vi "New.vi"(4 "Plugin":refnum<class "Plugin.lvclass">, 5 "thread base name":string="untitled", 6 "Logging Interface":refnum<class "Logging Interface.lvclass">, 7 "Plugin Interfaces Pool":refnum<class "Plugin Interface Pool.lvclass">, 8 "error in (no error)":errorcluster, 9 "Transfer Groups":refnum<class "Transfer Group.lvclass">[](array[class]), 10 "thread configuration":T1={"buffer converter settings"=[], "transceiver settings"=[], "custom settings"=[], "processor"=-2, "priority offset"=0}, 11 "Plugin Thread type":refnum<class "Plugin Thread.lvclass">) -> (0 "error out":errorcluster, 2 "Plugin Thread Interface":refnum<class "Plugin Interface.lvclass">, 3 "Plugin Thread out":refnum<class "Plugin Thread.lvclass">)   [LabVIEW 2017, in "DSF Core.lvlib" / "Plugin Thread.lvclass"]
uses:
  Thread/Plugin/Plugin Thread.lvclass
  C:/Git/DSF/Core/Classes/Thread/Thread.lvclass
  Transfer Group/Transfer Group.lvclass
  Pool/Plugin Interface/Plugin Interface Pool.lvclass
  Interface/Plugin/Plugin Interface.lvclass
  C:/Git/DSF/Core/Classes/Interface/Interface.lvclass
  Typedefs/DSF Engine Plugin Thread Configuration.ctl
  Typedefs/DSF Settings Info.ctl
  Interface/Logging/Logging Interface.lvclass
  Plugin/Plugin.lvclass
  Thread/Thread Settings.ctl
  Thread/Plugin/Plugin Thread.lvclass/Plugin Thread.ctl
  Thread/Thread.lvclass
  Interface/Interface.lvclass
  Timing/Timing.lvclass
  DSF Core.lvlib
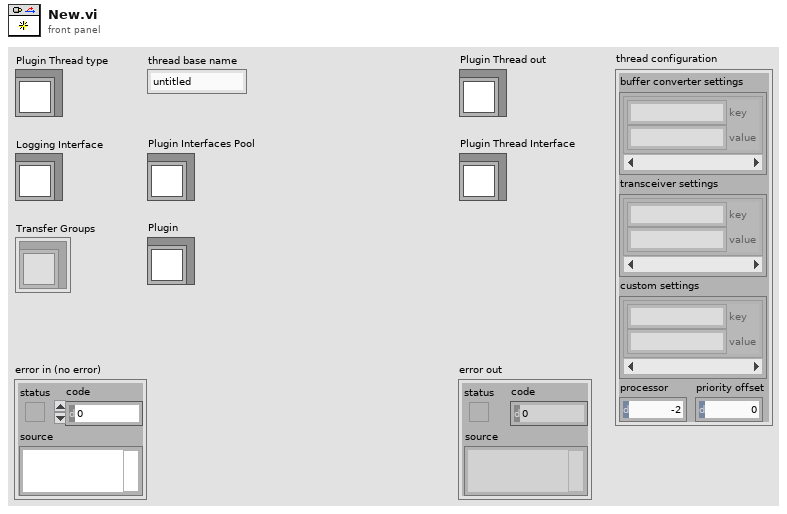
[diagram p1: front panel]
types:
  T1 = typedef "DSF Core.lvlib/DSF Engine Plugin Thread Configuration.ctl" = cluster{"buffer converter settings":T2, "transceiver settings":T2, "custom settings":T2, "processor":i32, "priority offset":i16}
  T2 = typedef "DSF Core.lvlib/DSF Settings Info.ctl" = cluster{"key":string, "value":string}[]
  T3 = typedef "DSF Core.lvlib/Thread.lvclass/Thread Settings.ctl" = cluster{"Priority":u16, "Processor":i32, "ID":i32}
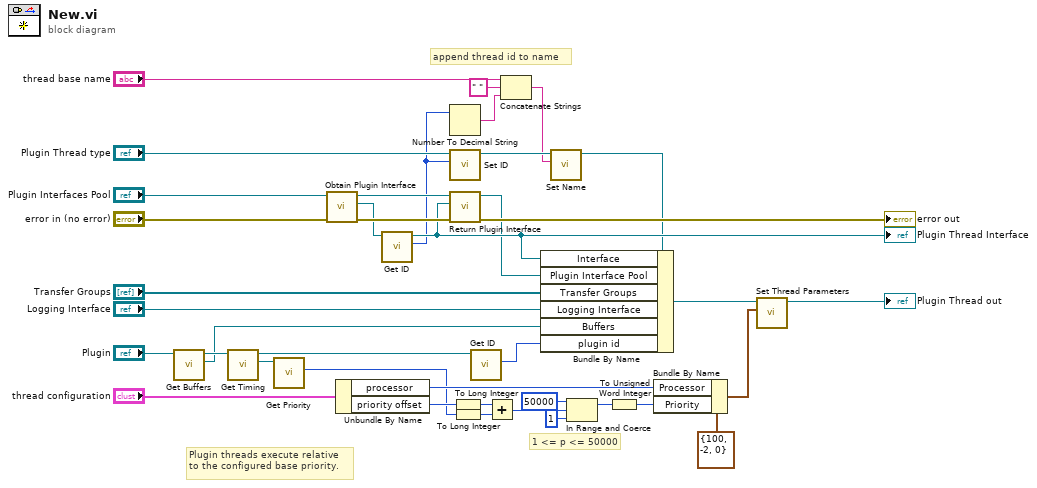
[diagram p0: block diagram]
diagram:
  # "1 <= p <= 50000"
  # "append thread id to name"
  # "Plugin threads execute relative to the configured base priority."
  n1 = call "Get Buffers.vi"("Plugin in"="Plugin") -> ("Buffers"=w5:refnum<class "Buffers.lvclass">, "Plugin out"=w6:refnum<class "Plugin.lvclass">)  [unwired: 9 in]
  n2 = call "Get Timing.vi"("Plugin in"=w6) -> ("Timing"=w8:refnum<class "Timing.lvclass">, "Plugin out"=w3:refnum<class "Plugin.lvclass">)  [unwired: 9 in]
  n3 = call "Get Priority.vi"("Timing in"=w8) -> ("Priority"=w4:u16)  [unwired: 9 in, 1 out]
  n4 = call "Obtain Plugin Interface.vi"("error in (no error)"="error in (no error)", "Plugin Interface Pool in"="Plugin Interfaces Pool") -> ("error out"=w38:errorcluster, "Plugin Interface"=w33:refnum<class "Plugin Interface.lvclass">, "Plugin Interface Pool out"=w32:refnum<class "Plugin Interface Pool.lvclass">)  [unwired: 6 in, 1 out]
  n5 = Unbundle By Name("thread configuration") -> ("processor"=w20:i32, "priority offset"=w21:i16)
  n6 = call "Get ID.vi"("Interface in"=w33) -> ("ID"=w11:i32, "Interface out"=w31:refnum<class "Plugin Interface.lvclass">)  [unwired: 9 in]
  "Plugin Thread Interface" <- w31
  n7 = Number To Decimal String(number=w11) -> (decimal integer string=w14:string)  [unwired: 1 in]
  n8 = call "Set ID.vi"("ID"=w11, "Thread in"="Plugin Thread type") -> ("Thread out"=w16:refnum<class "Plugin Thread.lvclass">)  [unwired: 9 in]
  n9 = call "Return Plugin Interface.vi"("error in (no error)"=w38, "Plugin Interface"=w31, "Plugin Interface Pool in"=w32) -> ("error out"=→"error out":errorcluster, "Plugin Interface Pool out"=w30:refnum<class "Plugin Interface Pool.lvclass">)  [unwired: 6 in, 1 out]
  n10 = To Long Integer(number=w21) -> (32bit integer=w28:i32)
  n11 = To Long Integer(number=w4) -> (32bit integer=w27:i32)
  n12 = call "Get ID.vi"("Plugin in"=w3) -> ("id"=w2:i32)  [unwired: 9 in, 1 out]
  n13 = Add(x=w28, y=w27) -> (x+y=w26:i32)
  n14 = Concatenate Strings("thread base name", " ", w14) -> (w10:string)
  n15 = call "Set Name.vi"("name"=w10, "Thread in"=w16) -> ("Thread out"=w15:refnum<class "Plugin Thread.lvclass">)  [unwired: 9 in]
  n16 = Bundle By Name(cluster=w15, "Interface"=w31, "Plugin Interface Pool"=w30, "Transfer Groups"="Transfer Groups", "Logging Interface"="Logging Interface", "Buffers"=w5, "plugin id"=w2) -> (w18:refnum<class "Plugin Thread.lvclass">)
  n17 = In Range and Coerce(upper limit=50000, x=w26, lower limit=1) -> (coerced(x)=w22:i32)  [unwired: 1 out]
  n18 = To Unsigned Word Integer(number=w22) -> (unsigned 16bit integer=w25:u16)
  n19 = Bundle By Name(cluster=T3 {"Priority"=100, "Processor"=-2, "ID"=0} ("thread settings"), "Processor"=w20, "Priority"=w25) -> (w17:T3)
  n20 = call "Set Thread Parameters.vi"("thread settings"=w17, "Thread in"=w18) -> ("Thread out"=→"Plugin Thread out":refnum<class "Plugin Thread.lvclass">)  [unwired: 9 in]
